vi "TestHB_Emb_2.vi"() -> ()   [LabVIEW 2012]
doc: "SciScan 1.2 160622"
uses:
  SubVIs/Master Slave messaging Flags.ctl
  Custom Controls and Typedefs/HB_Error Conditions Cluster.ctl
  Custom Controls and Typedefs/Heartbeat information cluster.ctl
  Custom Controls and Typedefs/Heartbeat Event Source.ctl
  Custom Controls/Heartbeat_States.ctl
  SubVIs/Heartbeat state manager Input VI names.ctl
  Custom Controls and Typedefs/HB Actionable Event.ctl
  Custom Controls and Typedefs/HFG Commands.ctl
panel:
  out "Master instr\nreceived":i32
  out "Slave conf\nreceived":i32
  out "Heartbeat information cluster":T1
  out "Error conditions Cluster":T4
  out "Master-Slave messaging Flags":T5={"Instruction available"=TRUE, "Slave action completed"=TRUE, "Slave Ready?"=FALSE}
  in  "stop":bool
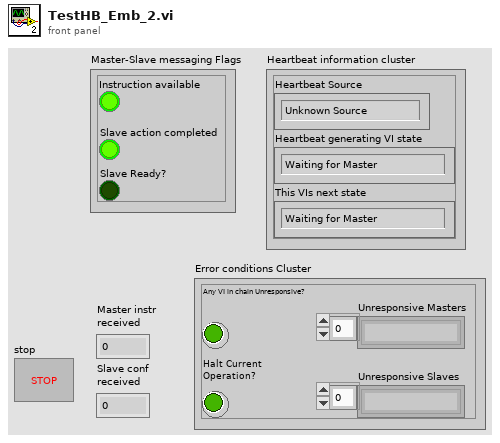
[diagram p1: front panel]
types:
  T1 = typedef "Heartbeat information cluster.ctl" = cluster{"Heartbeat Source":T2, "Heartbeat generating VI state":T3, "This VIs next state":T3}
  T2 = typedef "Heartbeat Event Source.ctl" = enum16{"Unknown Source", "Timeout", "This VI", "Master", "Slave"}
  T3 = typedef "Heartbeat_States.ctl" = enum16{"Waiting for Master", "Instruction Issued", "Waiting for Slave Completion", "Completed", "Cancelled", "Failed", "Broken Link"}
  T4 = typedef "HB_Error Conditions Cluster.ctl" = cluster{"Any VI in chain Unresponsive?":bool, "Halt Current Operation?":bool, "Unresponsive Masters":string[], "Unresponsive Slaves":string[]}
  T5 = typedef "Master Slave messaging Flags.ctl" = cluster{"Instruction available":bool, "Slave action completed":bool, "Slave Ready?":bool}
  T6 = typedef "HB Actionable Event.ctl" = enum16{"Master instruction event", "Slave ready event", "Slave unavailable event", "Cancelled or Failed event", "Slave action complete event", "QUIT", "Broken Link", "Recovered from Broken Link"}
  T7 = typedef "Heartbeat state manager Input VI names.ctl" = cluster{"Current VI name":string, "Master VI Names":string[], "Slave VI Names":string[]}
  T8 = typedef "HFG Commands.ctl" = enum16{"Set", "Get", "Initialize"}
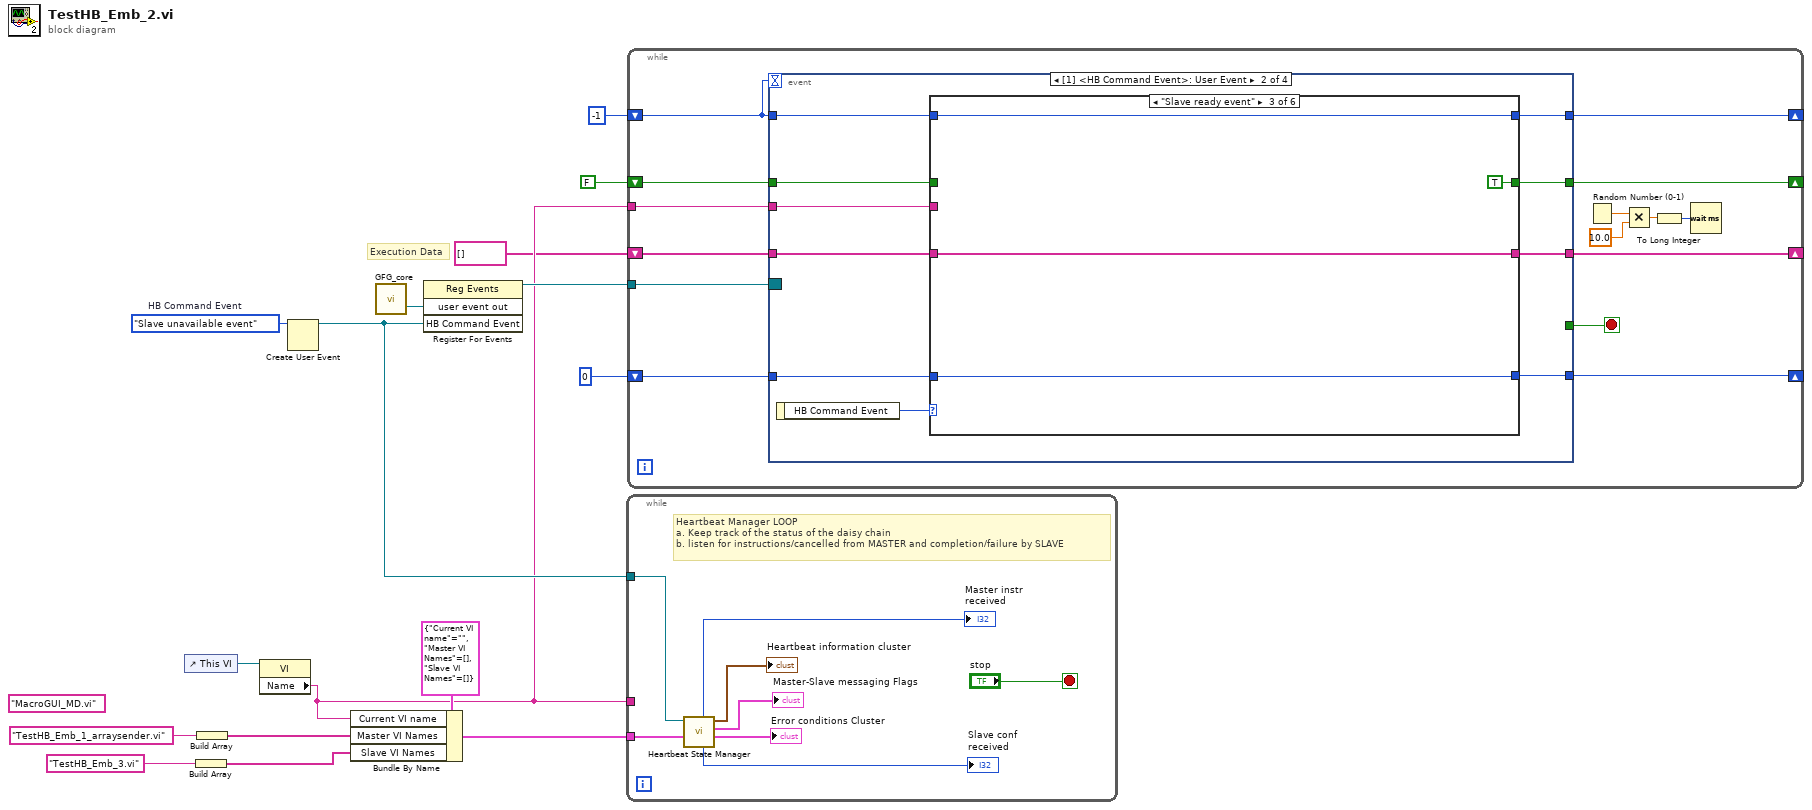
[diagram p0: block diagram]
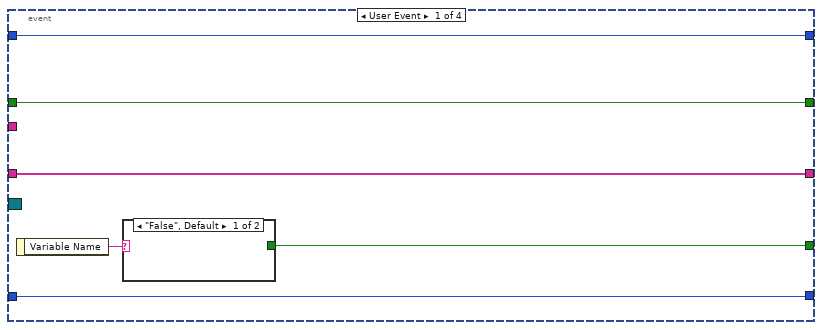
[diagram p2: hidden frame]
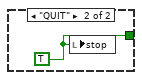
[diagram p3: hidden frame]
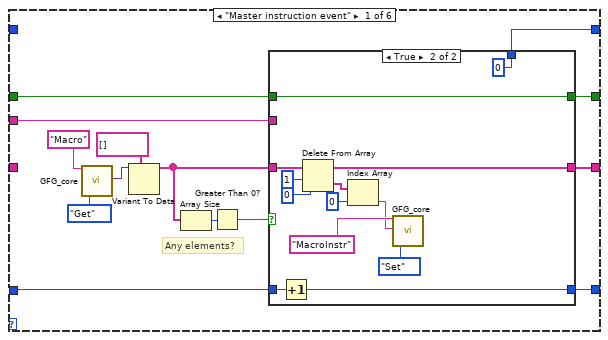
[diagram p4: hidden frame]
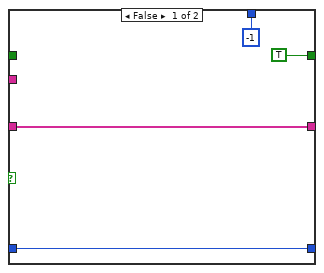
[diagram p5: hidden frame]
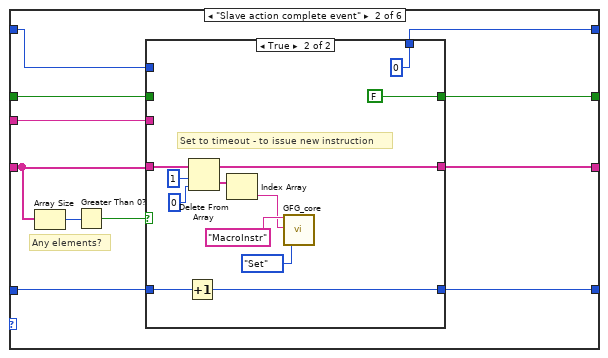
[diagram p6: hidden frame]
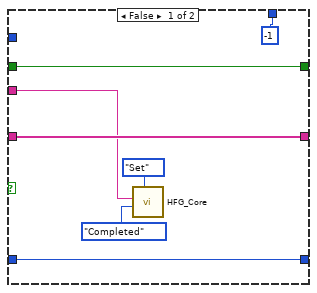
[diagram p7: hidden frame]
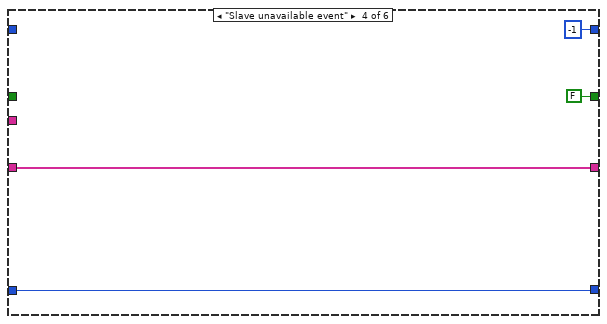
[diagram p8: hidden frame]
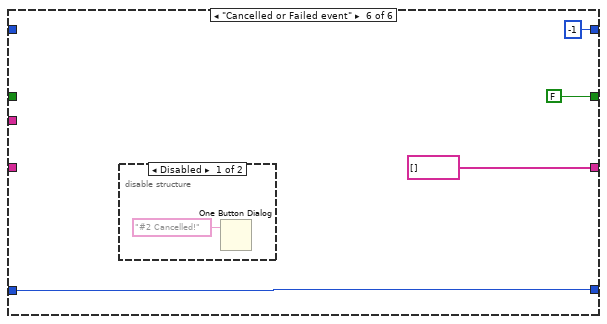
[diagram p10: hidden frame]
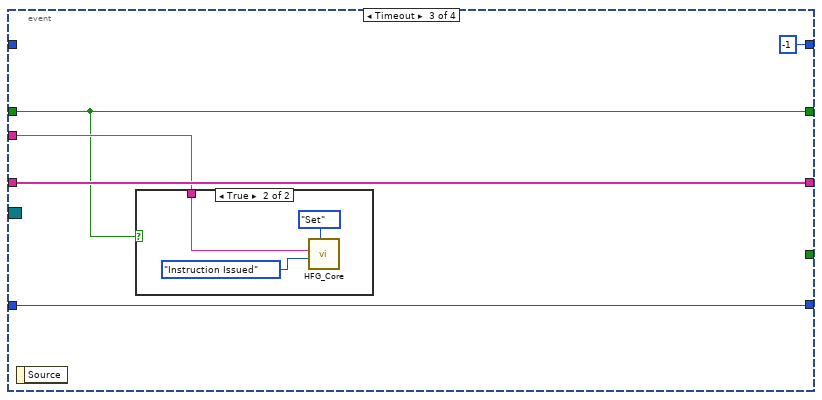
[diagram p12: hidden frame]
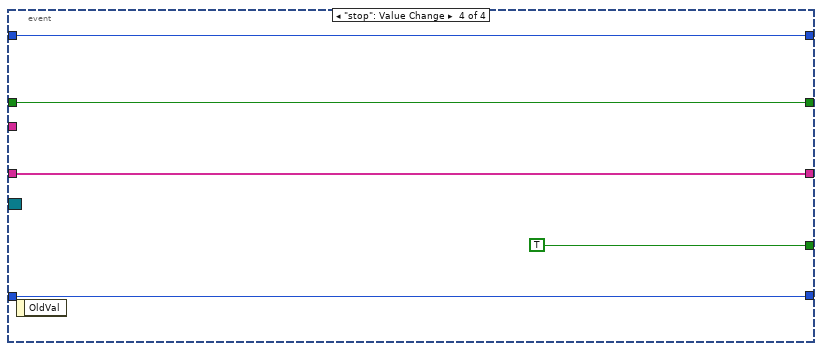
[diagram p14: hidden frame]
diagram:
  (unwired) "MacroGUI_MD.vi"
  w8 = HB_Actionable_Event."Slave unavailable event"  # HB Command Event
  # "Execution Data"
  n1 = control-ref of="This VI"() -> (w14:refnum<vi>)
  n2 = Build Array("TestHB_Emb_3.vi") -> (w11:string[])
  n3 = Build Array("TestHB_Emb_1_arraysender.vi") -> (w12:string[])
  n4 = property class="VI"(reference=w14) -> ("Name"=w6:string)  [unwired: 1 in, 2 out]
  n5 = Create User Event(user event datatype=w8) -> (user event=w7:refnum<user-event>)  [unwired: 1 in, 1 out]
  n6 = Bundle By Name(cluster=T7 {"Current VI name"="", "Master VI Names"=[], "Slave VI Names"=[]} ("Heartbeat state manager Input VI names 2"), "Current VI name"=w6, "Master VI Names"=w12, "Slave VI Names"=w11) -> (w13:T7)
  n7 = call "GFG_core.vi"() -> ("user event out"=w10:refnum<user-event>)  [unwired: 13 in, 6 out]
  n8 = register-events(w10, w7) -> (reference out=w9:refnum<event-registration>)  [unwired: 2 in, 1 out]
  n9 = while {
    tunnel: w13 -> [w24]
    tunnel: w6 -> [_]
    tunnel: w7 -> [w19]
    stop <- "stop" stop-if-true
    # "Heartbeat Manager LOOP \na. Keep track of the status of the daisy chain\nb. listen for instructions/cancelled from MASTER and completion/failure by SLAVE"
    n10 = call "Heartbeat State Manager.vi"("Heartbeat state manager Input VI names"=w24, "HB Command Event IN"=w19) -> ("Error conditions Cluster"=→"Error conditions Cluster":T4, "Master-Slave messaging Flags"=→"Master-Slave messaging Flags":T5, "Heartbeat information cluster"=→"Heartbeat information cluster":T1, "Slave Completions Received"=→"Slave conf\nreceived":i32, "Master Instructions Issued"=→"Master instr\nreceived":i32)  [unwired: 4 in, 1 out]
  }
  n11 = while {
    tunnel: w9 -> [w39]
    tunnel: w6 -> [w37]
    shift-right: [w34] -> _
    shift-left: string[] [] -> [w36]
    shift-right: [w33] -> _
    shift-left: 0 -> [w35]
    shift-right: [w31] -> _
    shift-left: FALSE ("slave ready") -> [w32]
    shift-right: [w25] -> _
    shift-left: -1 -> [w26]
    stop <- w38 stop-if-true
    n12 = event shown="[1] <HB Command Event>: User Event" {
      selector: w39 -> [_ _ _ _]
      dyn-events: _ -> [_ _ _ _]
      timeout: w26 -> [_ _ _ _]
      tunnel: [w44 _ _ TRUE] -> w38
      tunnel: w37 -> [_ w55 w137 _]
      tunnel: w36 -> [w43 w54 w138 w146]
      tunnel: w35 -> [w42 w53 w139 w145]
      tunnel: [w42 w52 w139 w145] -> w33
      tunnel: [w43 w51 w138 w146] -> w34
      tunnel: w32 -> [w41 w50 w135 w144]
      tunnel: [w41 w49 w135 w144] -> w31
      tunnel: w26 -> [w40 w47 _ w143]
      tunnel: [w40 w48 -1 w143] -> w25
      event User Event {
        n13 = event-data() -> ("Variable Name"=w45:string)  [unwired: 1 in]
        n14 = case shown="\"False\", Default" w45 {
          tunnel: [_ w46] -> w44
          frame "False", Default {
          }
          frame "QUIT" {
            w46 = TRUE
            n15 = local write "stop"(w46) -> ()
          }
        }
      }
      event User Event {
        n16 = event-data() -> ("HB Command Event"=w56:T6)  [unwired: 1 in]
        n17 = case shown="\"Slave ready event\"" w56 {
          tunnel: [w70 w95 w119 w124 w129 string[] []] -> w51
          tunnel: w54 -> [_ w93 w119 w124 w129 _]
          tunnel: w55 -> [w69 w92 _ _ _ _]
          tunnel: [w67 w94 w118 w123 w128 w132] -> w52
          tunnel: w53 -> [w68 w96 w118 w123 w128 w132]
          tunnel: [w66 w91 TRUE ("slave ready") FALSE ("slave ready") w127 FALSE ("slave ready")] -> w49
          tunnel: w50 -> [w57 w90 _ _ w127 _]
          tunnel: [w58 w89 w121 -1 w126 -1] -> w48
          tunnel: w47 -> [_ w88 w121 _ w126 _]
          frame "Master instruction event" {
            # "Any elements?"
            n18 = call "GFG_core.vi"("Variable Name in"="Macro", "Action"=enum16{"Init", "Set", "Get", "Clear"}."Get") -> ("Variant Out"=w63:variant)  [unwired: 11 in, 6 out]
            n19 = Variant To Data(type=string[] [], Variant=w63) -> (data=w60:string[])  [unwired: 1 in, 1 out]
            n20 = Array Size(array=w60) -> (size(s)=w61:i32)
            n21 = Greater Than 0?(x=w61) -> (x > 0?=w59:bool)
            n22 = case shown="True" w59 {
              tunnel: w60 -> [w74 w87]
              tunnel: [w74 w86] -> w70
              tunnel: w69 -> [_ _]
              tunnel: w68 -> [w73 w78]
              tunnel: [w73 w77] -> w67
              tunnel: [TRUE w75] -> w66
              tunnel: [-1 0] -> w58
              tunnel: w57 -> [_ w75]
              frame False {
              }
              frame True {
                n23 = Increment(x=w78) -> (x+1=w77:i32)
                n24 = Delete From Array(array=w87, length=1, index=0) -> (deleted portion=w81:string[], array with subset deleted=w86:string[])
                n25 = Index Array(array=w81, index=0) -> (element=w79:string)
                n26 = call "GFG_core.vi"("Variable Name in"="MacroInstr", "Variant in"=w79, "Action"=enum16{"Init", "Set", "Get", "Clear"}."Set") -> ()  [unwired: 10 in, 7 out]
              }
            }
          }
          frame "Slave action complete event" {
            # "Any elements?"
            n27 = Array Size(array=w93) -> (size(s)=w97:i32)
            n28 = Greater Than 0?(x=w97) -> (x > 0?=w98:bool)
            n29 = case shown="True" w98 {
              tunnel: w93 -> [w105 w117]
              tunnel: [w105 w116] -> w95
              tunnel: w92 -> [w101 _]
              tunnel: w96 -> [w102 w109]
              tunnel: [w102 w108] -> w94
              tunnel: [w100 FALSE] -> w91
              tunnel: w90 -> [w100 _]
              tunnel: [-1 0] -> w89
              tunnel: w88 -> [_ _]
              frame False {
                n30 = call "HFG_Core.vi"("HFG Commands"=HFG_Commands."Set", "Heartbeat state IN"=Heartbeat_States."Completed", "VI Name (Calling VIs name by default)"=w101) -> ()  [unwired: 5 in, 4 out]
              }
              frame True {
                # "Set to timeout - to issue new instruction"
                n31 = Increment(x=w109) -> (x+1=w108:i32)
                n32 = Delete From Array(array=w117, length=1, index=0) -> (deleted portion=w111:string[], array with subset deleted=w116:string[])
                n33 = Index Array(array=w111) -> (element=w110:string)  [unwired: 1 in]
                n34 = call "GFG_core.vi"("Variable Name in"="MacroInstr", "Variant in"=w110, "Action"=enum16{"Init", "Set", "Get", "Clear"}."Set") -> ()  [unwired: 10 in, 7 out]
              }
            }
          }
          frame "Slave ready event" {
          }
          frame "Slave unavailable event" {
          }
          frame Default {
          }
          frame "Cancelled or Failed event" {
            n35 = disable-structure shown="Disabled" {
              frame Disabled {
                n36 = One Button Dialog(message="#2 Cancelled!") -> ()  [unwired: 1 in, 1 out]
              }
              frame Enabled {
              }
            }
          }
        }
      }
      event Timeout {
        n37 = event-data() -> ()  [unwired: 1 in, 1 out]
        n38 = case shown="True" w135 {
          tunnel: w137 -> [_ w140]
          frame False {
          }
          frame True {
            n39 = call "HFG_Core.vi"("HFG Commands"=HFG_Commands."Set", "Heartbeat state IN"=Heartbeat_States."Instruction Issued", "VI Name (Calling VIs name by default)"=w140) -> ()  [unwired: 5 in, 4 out]
          }
        }
      }
      event "stop": Value Change {
        n40 = event-data() -> ()  [unwired: 1 in, 1 out]
      }
    }
    n41 = Random Number (0-1)() -> (number: 0 to 1=w30:dbl)
    n42 = Multiply(x=w30, y=10.0) -> (x*y=w28:dbl)
    n43 = To Long Integer(number=w28) -> (32bit integer=w27:i32)
    n44 = Wait (ms)(milliseconds to wait=w27) -> ()  [unwired: 1 out]
  }
